vi "PH_SRDG645.evt Call Set Channel Settings.vi"(0 "i ref in":refnum<vi>, 2 "Generator Instance":string="N/A", 3 "Channel to set":T1=1000 items=["T0", "T1", "A", "B", "C", "D", "E", "F", "G", "H"], 4 "Channel Settings":T2={"Delay [s]"=0.0, "relative to"=1000} {"relative to" items=["T0", "T1", "A", "B", "C", "D", "E", "F", "G", "H"]; "Delay [s]" format="%#_12p"}, 5 "error IO":errorcluster) -> (14 "i ref out":refnum<vi>, 19 "error out":errorcluster)   [LabVIEW 2014, in "PH_SRDG645.lvlib"]
doc: "This VI sends a simple event call."
uses:
  PH_SRDG645.lvlib
  PH_SRDG645.Channel Settings.ctl
  instr.lib/SRDG645/Driver/Channel.ctl
  CS_Core/CSSystem/CoreLib/CoreLib.int 2 byte array.vi
  CS_Core/CSSystem/CoreLib/CoreLib.double 2 byte array.vi
  CS_Core/CSSystem/CoreLib/CoreLib.lvlib
  CS_Core/BaseProcess/BaseProcess.lvlib
  instr.lib/SRDG645/Stanford Research DG645 - Driver.lvlib
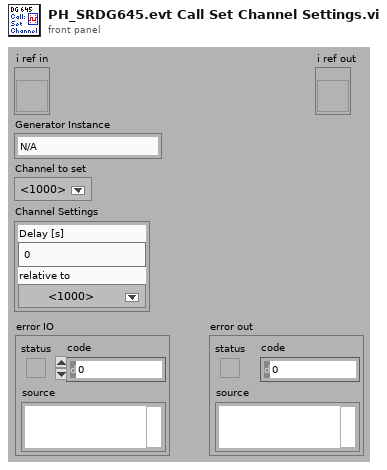
[diagram p1: front panel]
types:
  T1 = typedef "Stanford Research DG645 - Driver.lvlib/Channel.ctl" = i32
  T2 = typedef "PH_SRDG645.lvlib/PH_SRDG645.Channel Settings.ctl" = cluster{"Delay [s]":dbl, "relative to":i32}
  T3 = typedef "CoreDefs.rawDataType.ctl" = i8[]
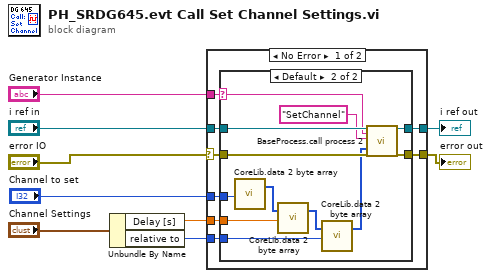
[diagram p0: block diagram]
diagram:
  n1 = Unbundle By Name("Channel Settings") -> ("Delay [s]"=w2:dbl, "relative to"=w3:i32)
  n2 = case shown="No Error" "error IO" {
    selector: "error IO" -> [w17 w32]
    tunnel: "Generator Instance" -> [w10 _]
    tunnel: [w16 w32] -> w9
    tunnel: [w14 w33] -> w8
    tunnel: w3 -> [w11 _]
    tunnel: w2 -> [w12 _]
    tunnel: "Channel to set" -> [w13 _]
    tunnel: "i ref in" -> [w15 w33]
    frame No Error {
      n3 = case shown="Default" w10 {
        selector: w10 -> [_ w24]
        tunnel: w17 -> [w18 w31]
        tunnel: [w18 w30] -> w16
        tunnel: w15 -> [w19 w29]
        tunnel: [w19 w28] -> w14
        tunnel: w13 -> [_ w22]
        tunnel: w12 -> [_ w20]
        tunnel: w11 -> [_ w23]
        frame "", "N/A" {
        }
        frame Default {
          n4 = call-poly "CoreLib.data 2 byte array.vi"("i32"=w22) -> ("byteArray out"=w26:T3)  [unwired: 18 in]
          n5 = call-poly "CoreLib.data 2 byte array.vi"("byteArray"=w26, "f64"=w20) -> ("byteArray out"=w25:T3)  [unwired: 17 in]
          n6 = call-poly "CoreLib.data 2 byte array.vi"("byteArray"=w25, "i32"=w23) -> ("byteArray out"=w21:T3)  [unwired: 17 in]
          n7 = call "BaseProcess.call process 2.vi"("i ref in"=w29, "Object"=w24, "Selector"="SetChannel", "Data"=w21, "error in (no error)"=w31) -> ("i ref out"=w28:refnum<vi>, "error out"=w30:errorcluster)  [unwired: 13 in]
        }
      }
    }
    frame Error {
    }
  }
  "error out" <- w9
  "i ref out" <- w8
